vi "transparent buttons.vi"(9 "control-level":string, 11 "Material-Scheme in":refnum<class "Material-Scheme.lvclass">) -> (1 "font color":u32(colorbox), 2 "colors array":cluster{"bg":u32, "fg":u32}[](array[cluster]))   [LabVIEW 2021, in "TSC Material Theme.lvlib" / "Material-Scheme.lvclass"]
doc: "application of the floating action button transparent buttons (text buttons) rules\n\nhttps://m3.material.io/components/buttons/specs#9c12a1a1-9a74-499c-8139-5cff551afe4f\n\n<b>Code Developed By:</b>\nTechnology Service Corporation\nwww.tsc.com/atcs\n\nDeveloper:\nDaniel Coons"
uses:
  Material-Scheme.lvclass
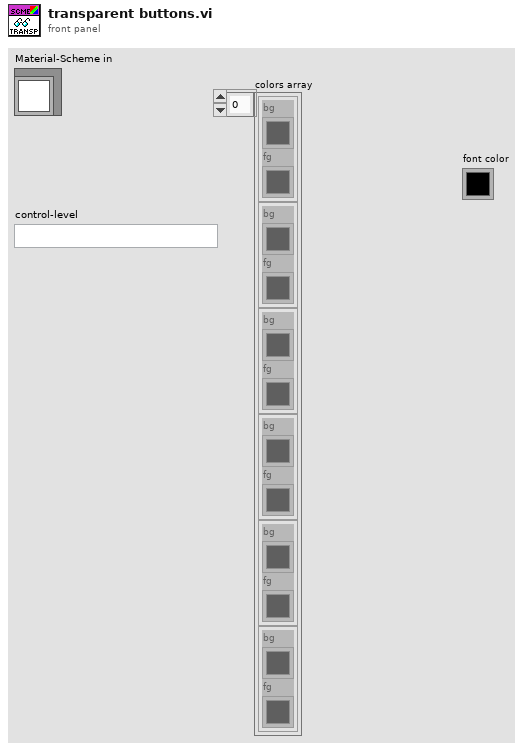
[diagram p1: front panel]
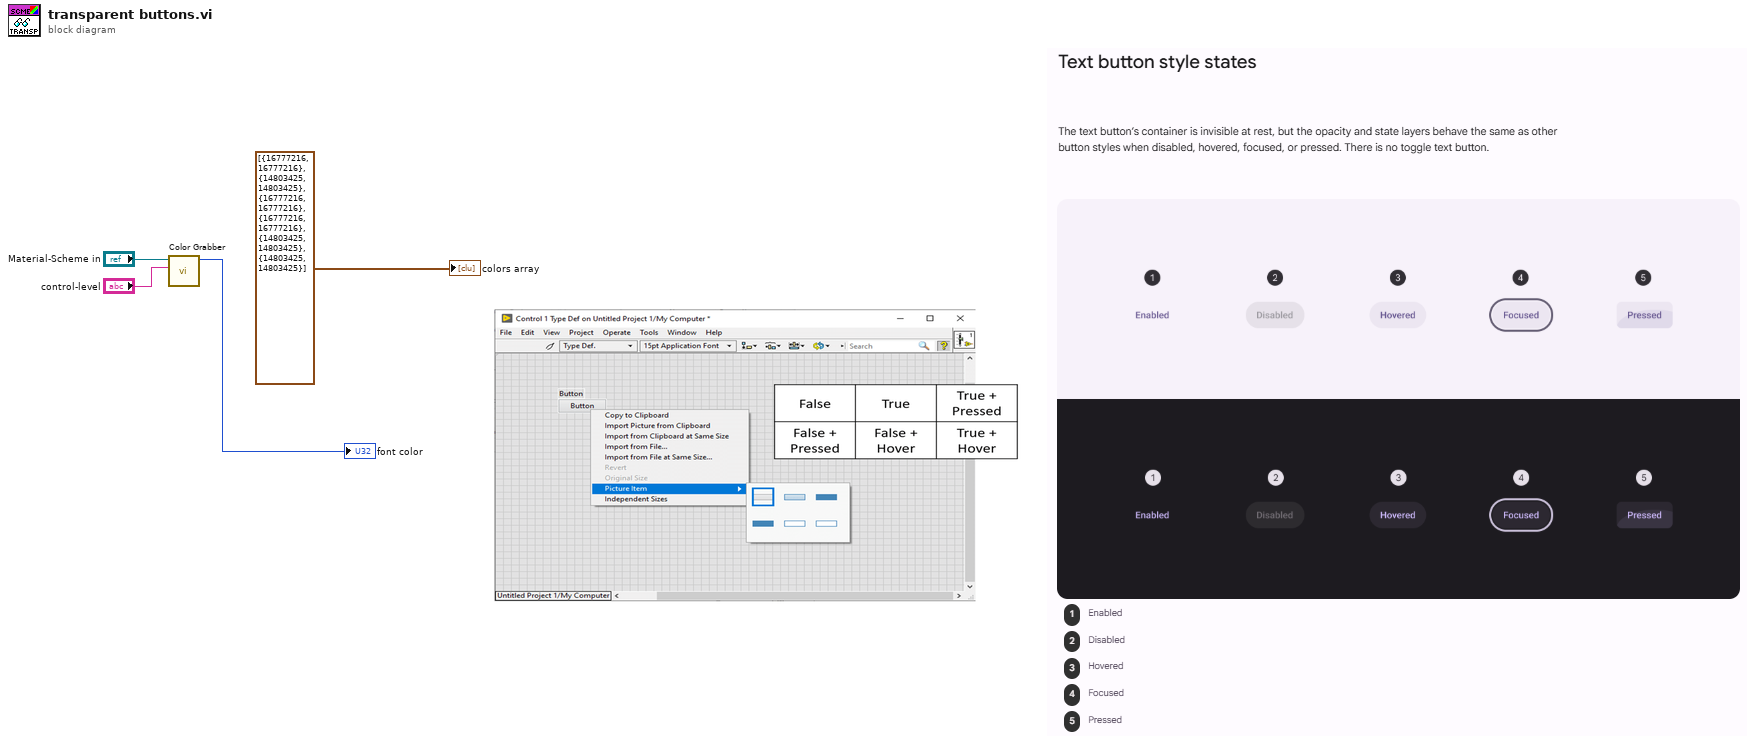
[diagram p0: block diagram]
diagram:
  n1 = call "Color Grabber.vi"("control-level"="control-level", "Material-Scheme in"="Material-Scheme in") -> ("color"=→"font color":u32)  [unwired: 3 in, 6 out]
  "colors array" <- cluster{"bg":u32, "fg":u32}[] [{"bg"=16777216, "fg"=16777216}, {"bg"=14803425, "fg"=14803425}, {"bg"=16777216, "fg"=16777216}, {"bg"=16777216, "fg"=16777216}, {"bg"=14803425, "fg"=14803425}, {"bg"=14803425, "fg"=14803425}] ("Colors Array")
